vi "Gather_Deal_Data_V2_0_20160104.vi"(8 "strModelChoice":string(combo)="WD5500", 9 "写指令":bool=TRUE, 10 "1号机端口":refnum<visa-resource-name>="COM1") -> (2 "缓冲区数据":u32=284, 3 "strResultArrayOut":string[](array[string]))   [LabVIEW 2011]
uses:
  <vilib>/Instr/_visa.llb/VISA Configure Serial Port (Instr).vi
panel:
  in  "Start":bool
  out "mu08BufSize":u8
  out "mbfDealData":bool
  out "mu08SendCmd":u8=3
  in  "CmdNumCount":u8
  out "mu08ArrayBuf0":u8[](array[numeric])=[90, 165, 142, 1, 240, 0, 1, 88, 200, 2, 0, 207, 3, 0, 219, 7, 1, 40, 11, 0, 0, 12, 0, 0, 13, 0, 0, 14, 0, 0, 21, 0, 0, 22, 0, 0, 23, 0, 0, 24, 150, 154, 29, 0, 0, 0, 0, 31, 0, 0, 33, 0, 34, 1, 64, 35, 0, 41, 0, 42, 0, 43, 0, 44, 12, 158, 45, 0, 0, 46, 0, 240, 47, 240, 48, 0, 49, 0, 50, 136, 51, 0, 52, 0, 53, 0, 54, 132, 58, 0, 59, 0, 60, 241, 61, 32, 32, 32, 32, 82, 64, 73, 83, 90, 2, 4, 0, 2, 4, 0, 0, 0, 0, 2, 0, 0, 0, 104, 201, 113, 49, 49, 53, 202, 70, 52, 48, 53, 203, 57, 48, 48, 66, 204, 32, 32, 48, 53, 251, 6, 87, 112, 90, 165, 142, 1, 240, 0, 1, 88, 200, 2, 0, 207, 3, 0, 219, 7, 1, 40, 11, 0, 0, 12, 0, 0, 13, 0, 0, 14, 0, 0, 21, 0, 0, 22, 0, 0, 23, 0, 0, 24, 150, 151, 29, 0, 0, 0, 0, 31, 0, 0, 33, 0, 34, 1, 64, 35, 0, 41, 0, 42, 0, 43, 0, 44, 12, 158, 45, 0, 0, 46, 0, 240, 47, 240, 48, 0, 49, 0, 50, 136, 51, 0, 52, 0, 53, 0, 54, 132, 58, 0, 59, 0, 60, 241, 61, 32, 32, 32, 32, 82, 64, 73, 83, 90, 2, 4, 0, 2, 4, 0, 0, 0, 0, 2, 0, 0, 0, 104, 201, 113, 49, 49, 53, 202, 70, 52, 48, 53, 203, 57, 48, 48, 66, 204, 32, 32, 48, 53, 251, 6, 95, 118] format="0x%x"
  out "mu16ArrayBuf0":u16=284
  out "mu08ArrayDatas":u8[](array[numeric])=[90, 165, 142, 1, 240, 0, 1, 88, 200, 2, 0, 207, 3, 0, 219, 7, 1, 40, 11, 0, 0, 12, 0, 0, 13, 0, 0, 14, 0, 0, 21, 0, 0, 22, 0, 0, 23, 0, 0, 24, 150, 154, 29, 0, 0, 0, 0, 31, 0, 0, 33, 0, 34, 1, 64, 35, 0, 41, 0, 42, 0, 43, 0, 44, 12, 158, 45, 0, 0, 46, 0, 240, 47, 240, 48, 0, 49, 0, 50, 136, 51, 0, 52, 0, 53, 0, 54, 132, 58, 0, 59, 0, 60, 241, 61, 32, 32, 32, 32, 82, 64, 73, 83, 90, 2, 4, 0, 2, 4, 0, 0, 0, 0, 2, 0, 0, 0, 104, 201, 113, 49, 49, 53, 202, 70, 52, 48, 53, 203, 57, 48, 48, 66, 204, 32, 32, 48, 53, 251, 6, 87, 112] format="0x%x"
  out "mu08ArrayDatasSize":u16=142
  out "命令":string
  in  "mbfUartClearOne":bool=TRUE
  out "Time":u32=400
  in  "Start_2":bool
  in  "CmdNumCount 2":u8
  out "strResultArrayOut 2":string[](array[string])
  out "mbfDealData 2":bool
  out "mu08SendCmd_2":u8=3
  in  "写指令_2":bool=TRUE
  out "Time_2":u32=400
  out "缓冲区数据_2":u32=284
  out "mu08ArrayBuf0 2":u8[](array[numeric])=[90, 165, 142, 1, 240, 0, 1, 88, 200, 2, 0, 207, 3, 0, 219, 7, 1, 40, 11, 0, 0, 12, 0, 0, 13, 0, 0, 14, 0, 0, 21, 0, 0, 22, 0, 0, 23, 0, 0, 24, 150, 154, 29, 0, 0, 0, 0, 31, 0, 0, 33, 0, 34, 1, 64, 35, 0, 41, 0, 42, 0, 43, 0, 44, 12, 158, 45, 0, 0, 46, 0, 240, 47, 240, 48, 0, 49, 0, 50, 136, 51, 0, 52, 0, 53, 0, 54, 132, 58, 0, 59, 0, 60, 241, 61, 32, 32, 32, 32, 82, 64, 73, 83, 90, 2, 4, 0, 2, 4, 0, 0, 0, 0, 2, 0, 0, 0, 104, 201, 113, 49, 49, 53, 202, 70, 52, 48, 53, 203, 57, 48, 48, 66, 204, 32, 32, 48, 53, 251, 6, 87, 112, 90, 165, 142, 1, 240, 0, 1, 88, 200, 2, 0, 207, 3, 0, 219, 7, 1, 40, 11, 0, 0, 12, 0, 0, 13, 0, 0, 14, 0, 0, 21, 0, 0, 22, 0, 0, 23, 0, 0, 24, 150, 151, 29, 0, 0, 0, 0, 31, 0, 0, 33, 0, 34, 1, 64, 35, 0, 41, 0, 42, 0, 43, 0, 44, 12, 158, 45, 0, 0, 46, 0, 240, 47, 240, 48, 0, 49, 0, 50, 136, 51, 0, 52, 0, 53, 0, 54, 132, 58, 0, 59, 0, 60, 241, 61, 32, 32, 32, 32, 82, 64, 73, 83, 90, 2, 4, 0, 2, 4, 0, 0, 0, 0, 2, 0, 0, 0, 104, 201, 113, 49, 49, 53, 202, 70, 52, 48, 53, 203, 57, 48, 48, 66, 204, 32, 32, 48, 53, 251, 6, 95, 118] format="0x%x"
  out "mu16ArrayBuf0_2":u16=284
  out "mu08ArrayDatas_2":u8[](array[numeric])=[90, 165, 142, 1, 240, 0, 1, 88, 200, 2, 0, 207, 3, 0, 219, 7, 1, 40, 11, 0, 0, 12, 0, 0, 13, 0, 0, 14, 0, 0, 21, 0, 0, 22, 0, 0, 23, 0, 0, 24, 150, 154, 29, 0, 0, 0, 0, 31, 0, 0, 33, 0, 34, 1, 64, 35, 0, 41, 0, 42, 0, 43, 0, 44, 12, 158, 45, 0, 0, 46, 0, 240, 47, 240, 48, 0, 49, 0, 50, 136, 51, 0, 52, 0, 53, 0, 54, 132, 58, 0, 59, 0, 60, 241, 61, 32, 32, 32, 32, 82, 64, 73, 83, 90, 2, 4, 0, 2, 4, 0, 0, 0, 0, 2, 0, 0, 0, 104, 201, 113, 49, 49, 53, 202, 70, 52, 48, 53, 203, 57, 48, 48, 66, 204, 32, 32, 48, 53, 251, 6, 87, 112] format="0x%x"
  out "mu08ArrayDatasSize_2":u16=142
  out "mu08BufSize_2":u8
  in  "strModelChoice_2":string(combo)="WD5500"
  out "命令_2":string
  in  "mbfUartClearOne 2":bool=TRUE
  in  "2号机端口":refnum<visa-resource-name>="COM3"
  in  "Start_3":bool
  out "命令_3":string
  in  "CmdNumCount_3":u8
  out "mu16ArrayBuf0_3":u16=284
  out "mu08ArrayDatasSize_3":u16=142
  out "mu08BufSize_3":u8
  out "mu08ArrayBuf0_3":u8[](array[numeric])=[90, 165, 142, 1, 240, 0, 1, 88, 200, 2, 0, 207, 3, 0, 219, 7, 1, 40, 11, 0, 0, 12, 0, 0, 13, 0, 0, 14, 0, 0, 21, 0, 0, 22, 0, 0, 23, 0, 0, 24, 150, 154, 29, 0, 0, 0, 0, 31, 0, 0, 33, 0, 34, 1, 64, 35, 0, 41, 0, 42, 0, 43, 0, 44, 12, 158, 45, 0, 0, 46, 0, 240, 47, 240, 48, 0, 49, 0, 50, 136, 51, 0, 52, 0, 53, 0, 54, 132, 58, 0, 59, 0, 60, 241, 61, 32, 32, 32, 32, 82, 64, 73, 83, 90, 2, 4, 0, 2, 4, 0, 0, 0, 0, 2, 0, 0, 0, 104, 201, 113, 49, 49, 53, 202, 70, 52, 48, 53, 203, 57, 48, 48, 66, 204, 32, 32, 48, 53, 251, 6, 87, 112, 90, 165, 142, 1, 240, 0, 1, 88, 200, 2, 0, 207, 3, 0, 219, 7, 1, 40, 11, 0, 0, 12, 0, 0, 13, 0, 0, 14, 0, 0, 21, 0, 0, 22, 0, 0, 23, 0, 0, 24, 150, 151, 29, 0, 0, 0, 0, 31, 0, 0, 33, 0, 34, 1, 64, 35, 0, 41, 0, 42, 0, 43, 0, 44, 12, 158, 45, 0, 0, 46, 0, 240, 47, 240, 48, 0, 49, 0, 50, 136, 51, 0, 52, 0, 53, 0, 54, 132, 58, 0, 59, 0, 60, 241, 61, 32, 32, 32, 32, 82, 64, 73, 83, 90, 2, 4, 0, 2, 4, 0, 0, 0, 0, 2, 0, 0, 0, 104, 201, 113, 49, 49, 53, 202, 70, 52, 48, 53, 203, 57, 48, 48, 66, 204, 32, 32, 48, 53, 251, 6, 95, 118] format="0x%x"
  out "缓冲区数据_3":u32=284
  out "mu08ArrayDatas_3":u8[](array[numeric])=[90, 165, 142, 1, 240, 0, 1, 88, 200, 2, 0, 207, 3, 0, 219, 7, 1, 40, 11, 0, 0, 12, 0, 0, 13, 0, 0, 14, 0, 0, 21, 0, 0, 22, 0, 0, 23, 0, 0, 24, 150, 154, 29, 0, 0, 0, 0, 31, 0, 0, 33, 0, 34, 1, 64, 35, 0, 41, 0, 42, 0, 43, 0, 44, 12, 158, 45, 0, 0, 46, 0, 240, 47, 240, 48, 0, 49, 0, 50, 136, 51, 0, 52, 0, 53, 0, 54, 132, 58, 0, 59, 0, 60, 241, 61, 32, 32, 32, 32, 82, 64, 73, 83, 90, 2, 4, 0, 2, 4, 0, 0, 0, 0, 2, 0, 0, 0, 104, 201, 113, 49, 49, 53, 202, 70, 52, 48, 53, 203, 57, 48, 48, 66, 204, 32, 32, 48, 53, 251, 6, 87, 112] format="0x%x"
  in  "strModelChoice 2":string(combo)="WD5500"
  in  "写指令_3":bool=TRUE
  in  "3号机端口":refnum<visa-resource-name>="COM3"
  in  "mbfUartClearOne_3":bool=TRUE
  out "mbfDealData_3":bool
  out "Time_3":u32=400
  out "strResultArrayOut_3":string[](array[string])
  out "mu08SendCmd_2 2":u8=3
  in  "Start_4":bool
  in  "strModelChoice_4":string(combo)="WD5500"
  out "Time_4":u32=400
  out "mbfDealData_4":bool
  in  "mbfUartClearOne_4":bool=TRUE
  out "strResultArrayOut_4":string[](array[string])
  out "mu08SendCmd_4":u8=3
  out "命令_4":string
  in  "写指令_4":bool=TRUE
  out "mu08ArrayDatas_4":u8[](array[numeric])=[90, 165, 142, 1, 240, 0, 1, 88, 200, 2, 0, 207, 3, 0, 219, 7, 1, 40, 11, 0, 0, 12, 0, 0, 13, 0, 0, 14, 0, 0, 21, 0, 0, 22, 0, 0, 23, 0, 0, 24, 150, 154, 29, 0, 0, 0, 0, 31, 0, 0, 33, 0, 34, 1, 64, 35, 0, 41, 0, 42, 0, 43, 0, 44, 12, 158, 45, 0, 0, 46, 0, 240, 47, 240, 48, 0, 49, 0, 50, 136, 51, 0, 52, 0, 53, 0, 54, 132, 58, 0, 59, 0, 60, 241, 61, 32, 32, 32, 32, 82, 64, 73, 83, 90, 2, 4, 0, 2, 4, 0, 0, 0, 0, 2, 0, 0, 0, 104, 201, 113, 49, 49, 53, 202, 70, 52, 48, 53, 203, 57, 48, 48, 66, 204, 32, 32, 48, 53, 251, 6, 87, 112] format="0x%x"
  in  "CmdNumCount_4":u8
  out "缓冲区数据_4":u32=284
  out "mu08BufSize_4":u8
  out "mu08ArrayBuf0_4":u8[](array[numeric])=[90, 165, 142, 1, 240, 0, 1, 88, 200, 2, 0, 207, 3, 0, 219, 7, 1, 40, 11, 0, 0, 12, 0, 0, 13, 0, 0, 14, 0, 0, 21, 0, 0, 22, 0, 0, 23, 0, 0, 24, 150, 154, 29, 0, 0, 0, 0, 31, 0, 0, 33, 0, 34, 1, 64, 35, 0, 41, 0, 42, 0, 43, 0, 44, 12, 158, 45, 0, 0, 46, 0, 240, 47, 240, 48, 0, 49, 0, 50, 136, 51, 0, 52, 0, 53, 0, 54, 132, 58, 0, 59, 0, 60, 241, 61, 32, 32, 32, 32, 82, 64, 73, 83, 90, 2, 4, 0, 2, 4, 0, 0, 0, 0, 2, 0, 0, 0, 104, 201, 113, 49, 49, 53, 202, 70, 52, 48, 53, 203, 57, 48, 48, 66, 204, 32, 32, 48, 53, 251, 6, 87, 112, 90, 165, 142, 1, 240, 0, 1, 88, 200, 2, 0, 207, 3, 0, 219, 7, 1, 40, 11, 0, 0, 12, 0, 0, 13, 0, 0, 14, 0, 0, 21, 0, 0, 22, 0, 0, 23, 0, 0, 24, 150, 151, 29, 0, 0, 0, 0, 31, 0, 0, 33, 0, 34, 1, 64, 35, 0, 41, 0, 42, 0, 43, 0, 44, 12, 158, 45, 0, 0, 46, 0, 240, 47, 240, 48, 0, 49, 0, 50, 136, 51, 0, 52, 0, 53, 0, 54, 132, 58, 0, 59, 0, 60, 241, 61, 32, 32, 32, 32, 82, 64, 73, 83, 90, 2, 4, 0, 2, 4, 0, 0, 0, 0, 2, 0, 0, 0, 104, 201, 113, 49, 49, 53, 202, 70, 52, 48, 53, 203, 57, 48, 48, 66, 204, 32, 32, 48, 53, 251, 6, 95, 118] format="0x%x"
  in  "4号机端口":refnum<visa-resource-name>="COM3"
  out "mu08ArrayDatasSize_4":u16=142
  out "mu16ArrayBuf0_4":u16=284
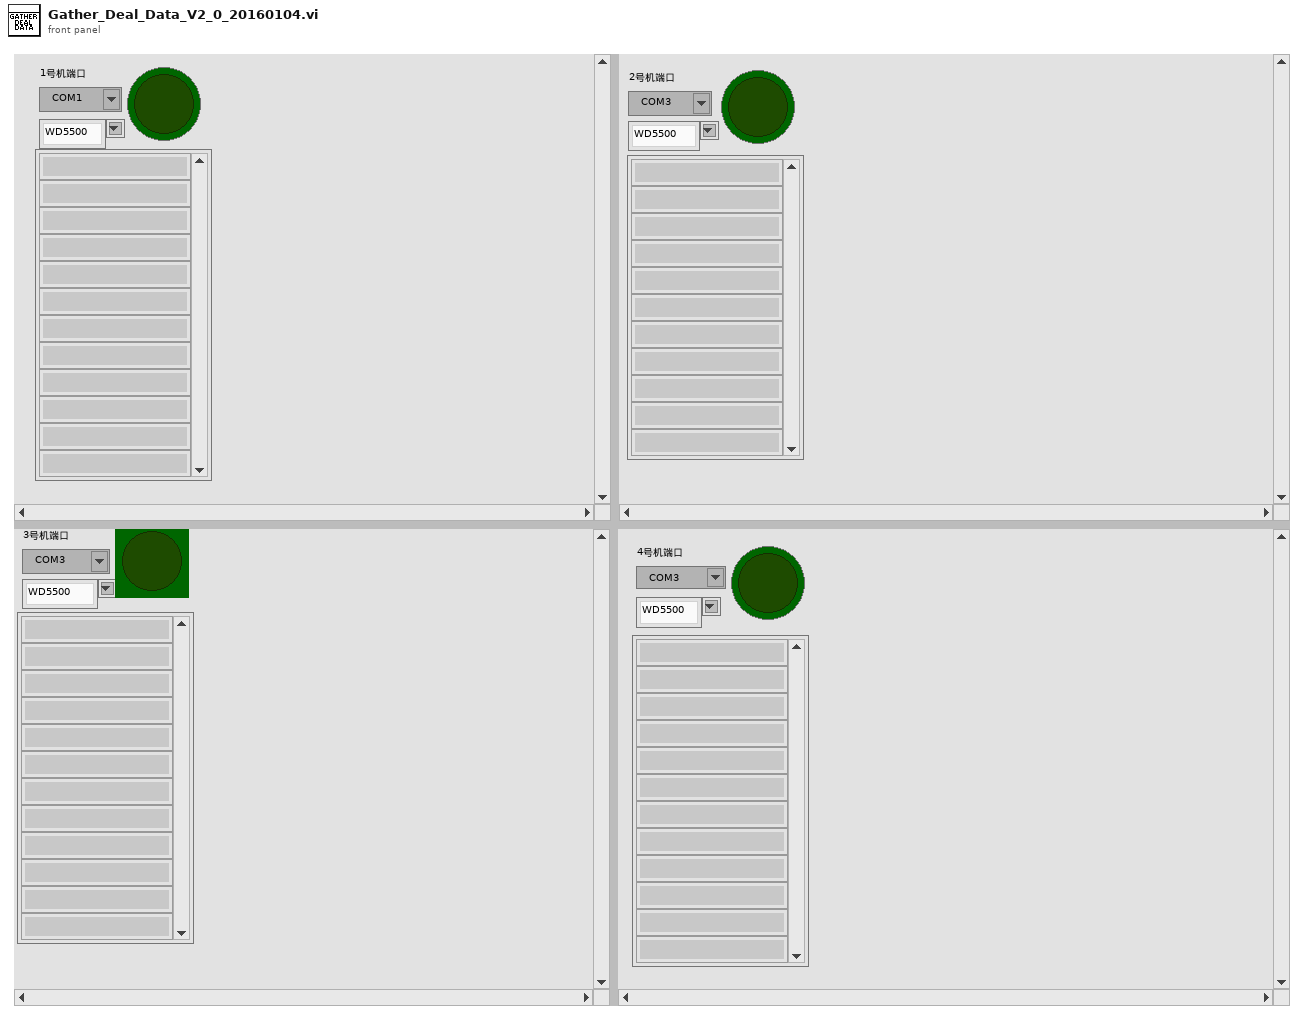
[diagram p1: front panel]
types:
  T1 = enum16{"open", "replace", "create", "open or create", "replace or create", "replace or create with confirmation"}
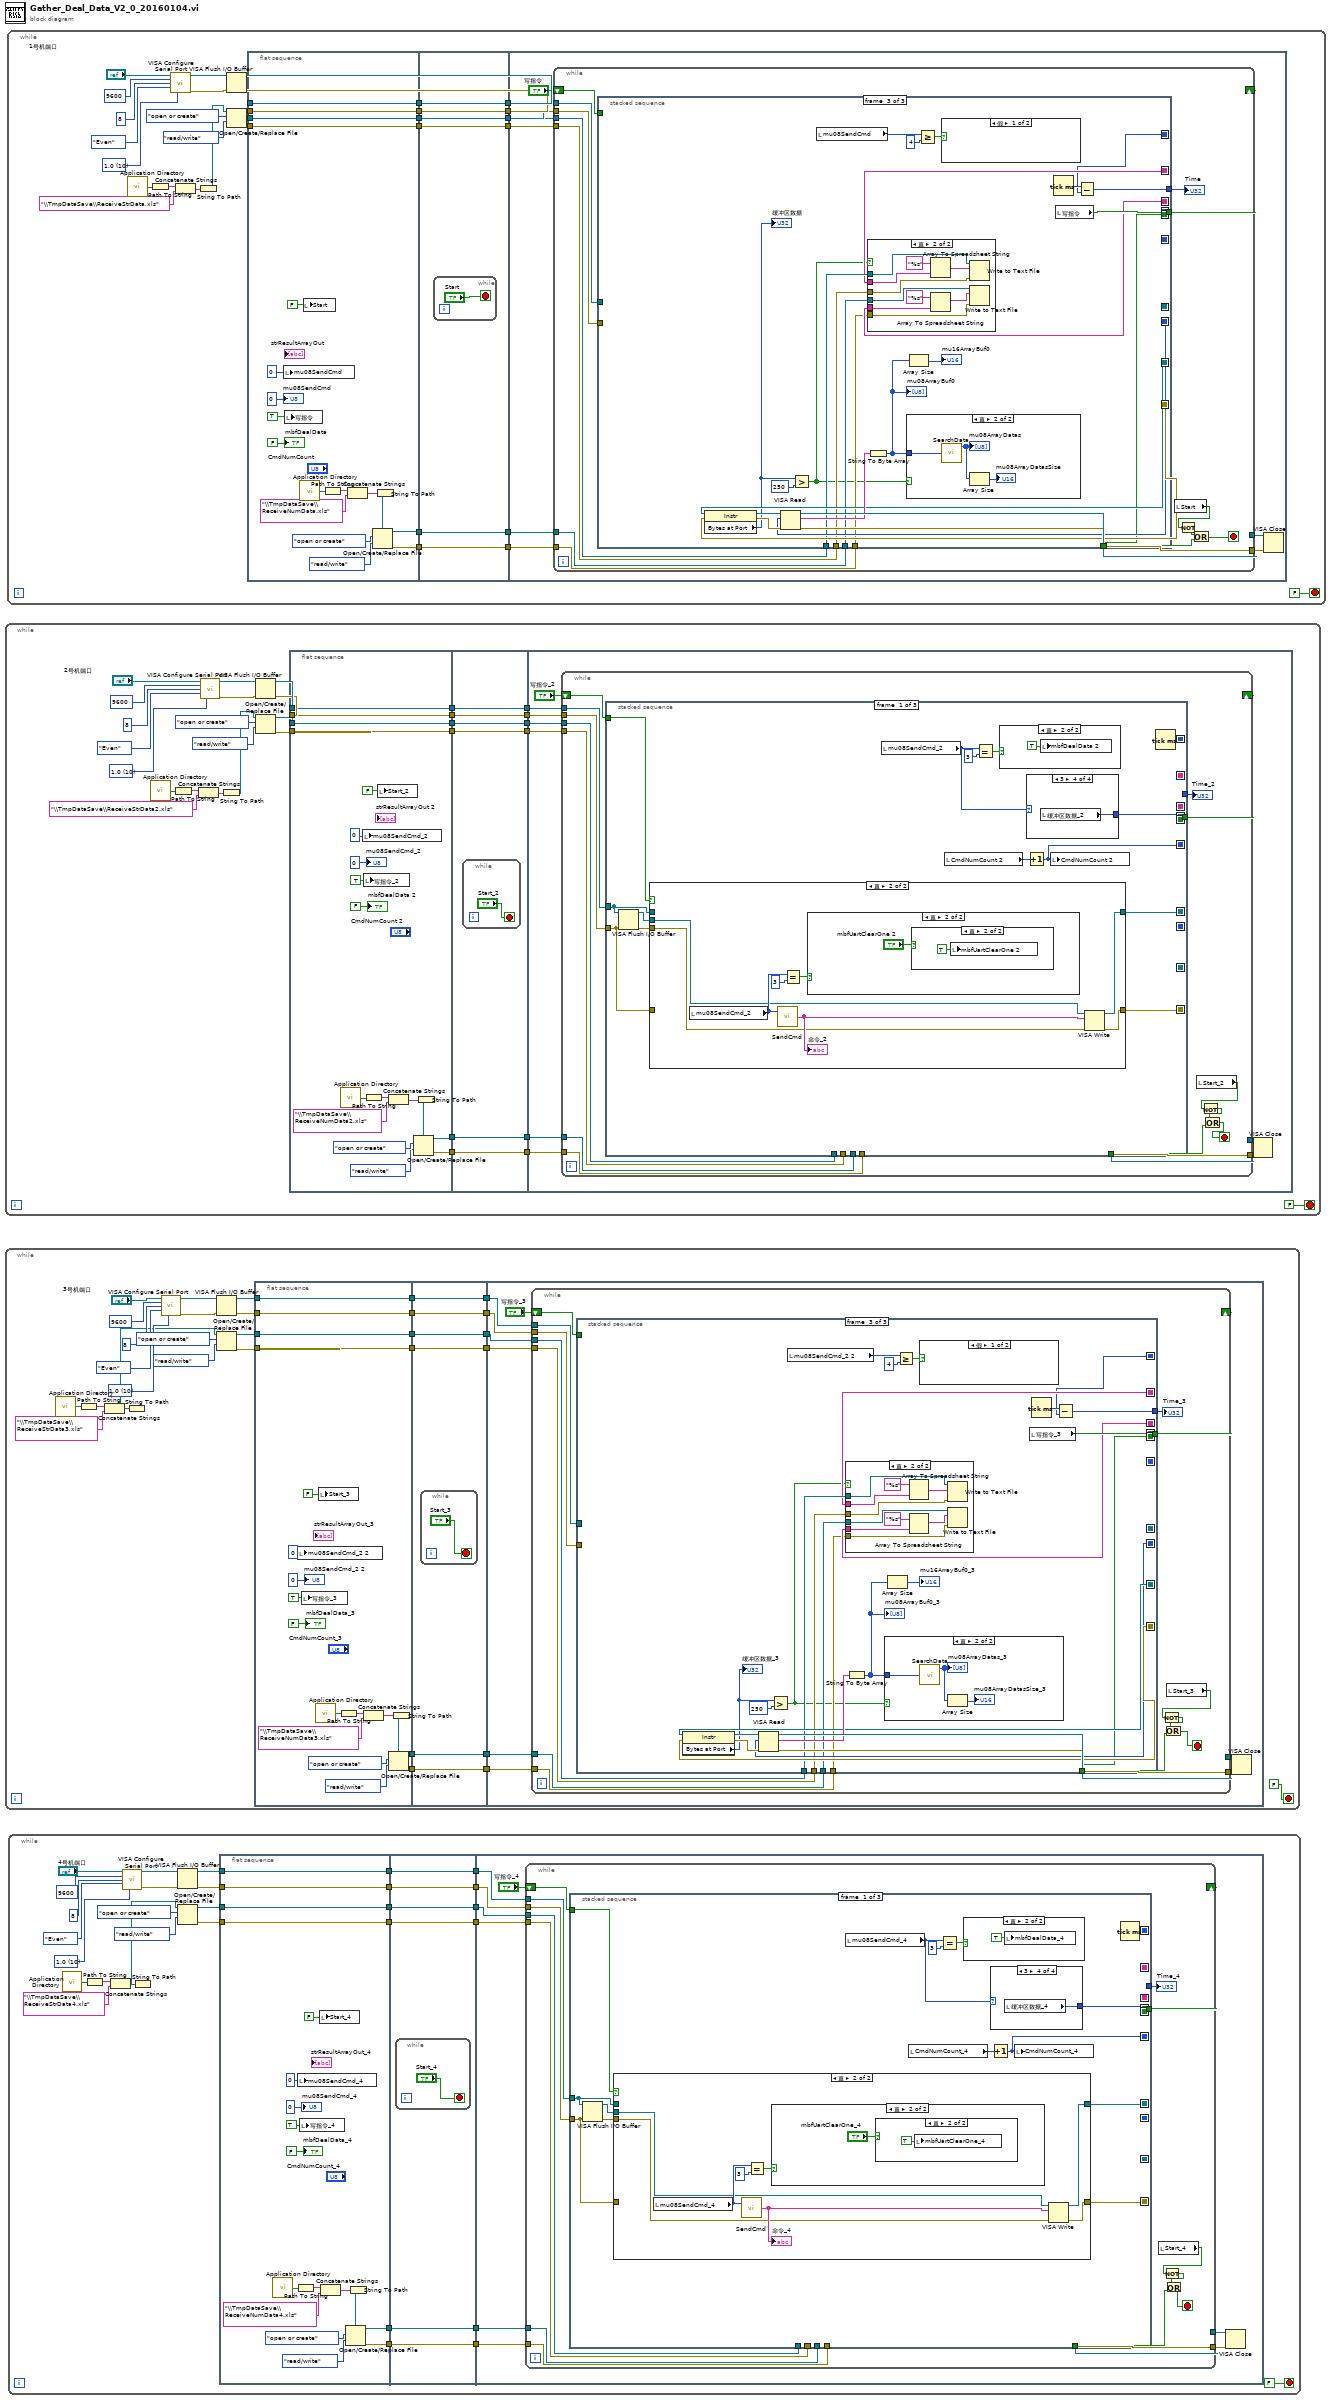
[diagram p0: block diagram]
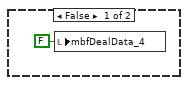
[diagram p2: hidden frame]
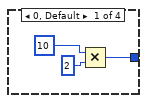
[diagram p3: hidden frame]
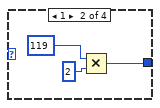
[diagram p4: hidden frame]
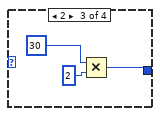
[diagram p5: hidden frame]
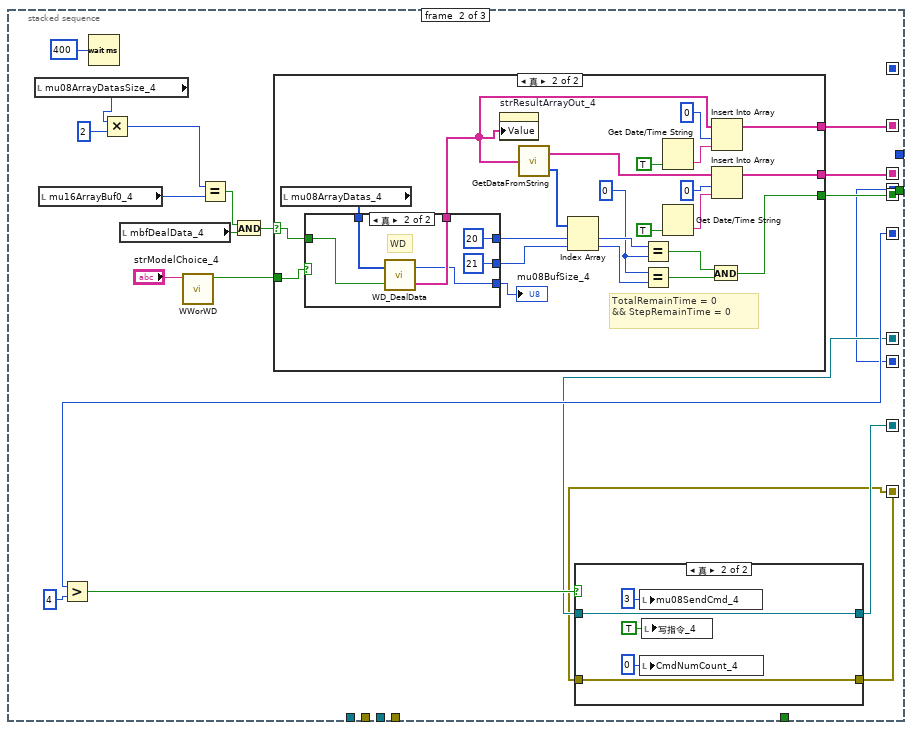
[diagram p9: hidden frame]
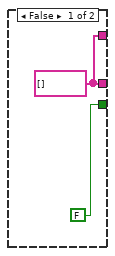
[diagram p10: hidden frame]
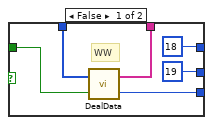
[diagram p11: hidden frame]
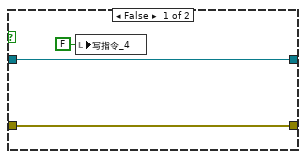
[diagram p12: hidden frame]
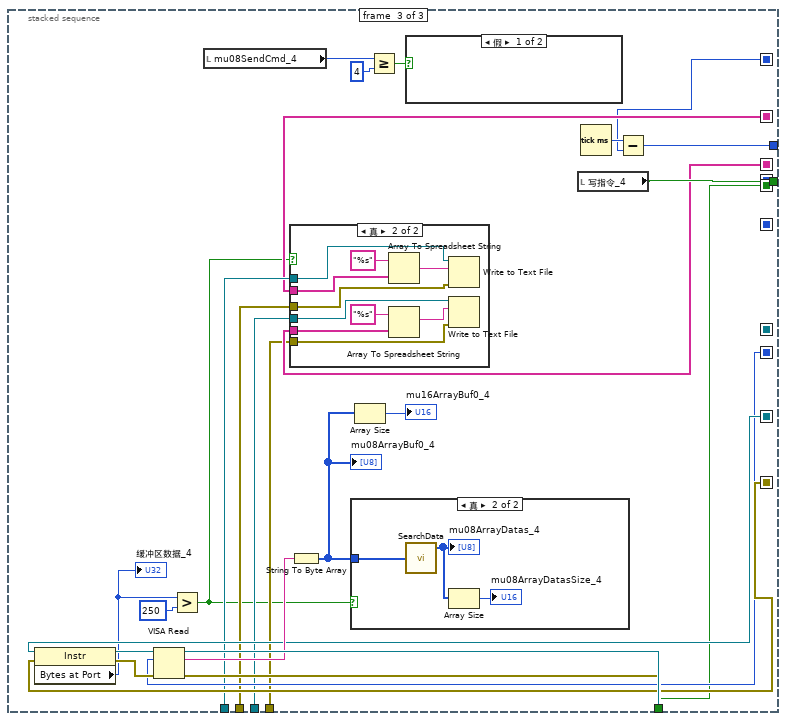
[diagram p13: hidden frame]
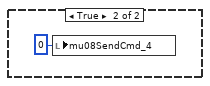
[diagram p16: hidden frame]
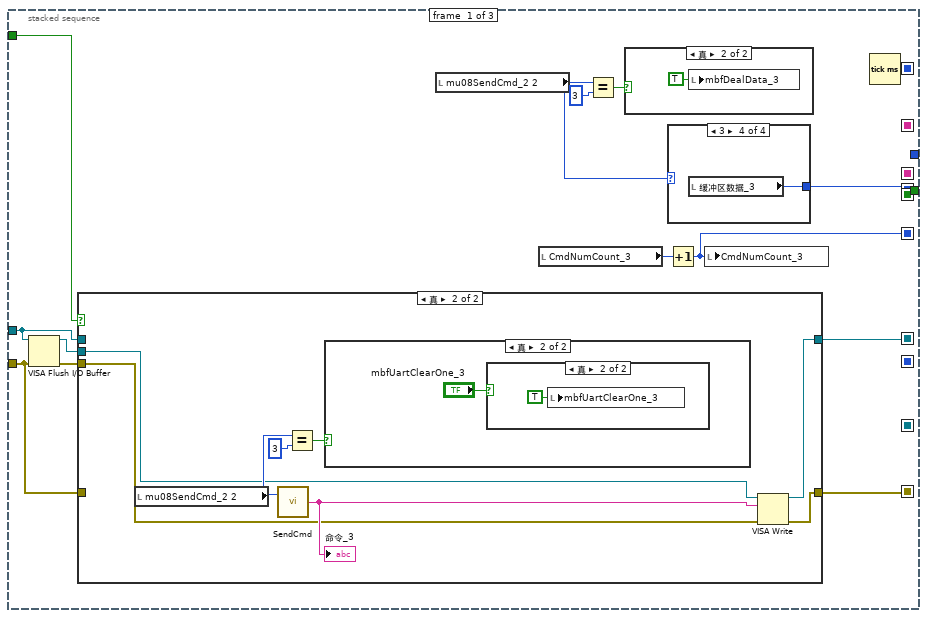
[diagram p17: hidden frame]
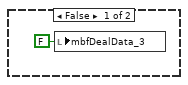
[diagram p18: hidden frame]
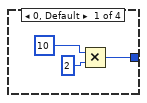
[diagram p19: hidden frame]
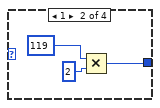
[diagram p20: hidden frame]
diagram:
  n1 = while {
    stop <- FALSE stop-if-true
    w15 = u16 10 items=["1.0"=10, "1.5"=15, "2.0"=20] ("stop bits (10: 1 bit)")
    n2 = call <vilib>:"Application Directory.vi"() -> ("Application Directory"=w5:path)
    n3 = Path To String(path=w5) -> (string=w4:string)
    n4 = Concatenate Strings(w4, "\\TmpDataSave\\ReceiveStrData2.xls" ("字符串")) -> (w2:string)
    n5 = call-poly "VISA Configure Serial Port"("VISA resource name"="2号机端口", "baud rate (9600)"=u32 9600, "data bits (8)"=u16 8, "parity (0:none)"=enum16{"None", "Odd", "Even", "Mark", "Space"}."Even", "stop bits (10: 1 bit)"=w15) -> ("VISA resource name out"=w14:refnum<visa-resource-name>, "error out"=w13:errorcluster)  [unwired: 9 in]
    n6 = String To Path(string=w2) -> (path=w8:path)
    n7 = VISA Flush I/O Buffer(VISA resource name=w14, error in (no error)=w13) -> (VISA resource name out=w12:refnum<visa-resource-name>, error out=w11:errorcluster)  [unwired: 1 in]
    n8 = Open/Create/Replace File(file path (use dialog)=w8, operation (0:open)=T1."open or create" ("操作(0:open)"), access (0:read/write)=enum16{"read/write", "read-only", "write-only"}."read/write" ("权限(0:read/write)")) -> (refnum out=w7:refnum<file>, error out=w6:errorcluster)  [unwired: 3 in, 1 out]
    n9 = flat-sequence {
      tunnel: w6 -> [w46]
      tunnel: w7 -> [w47]
      tunnel: w11 -> [w48]
      tunnel: w12 -> [w49]
      tunnel: [w49] -> w31
      tunnel: [w48] -> w30
      tunnel: [w47] -> w29
      tunnel: [w46] -> w28
      tunnel: [w33] -> w27
      tunnel: [w32] -> w26
      tunnel: [w55] -> w25
      tunnel: [w54] -> w24
      tunnel: [w53] -> w23
      tunnel: [w52] -> w22
      tunnel: [w51] -> w21
      tunnel: [w50] -> w20
      tunnel: w31 -> [w55]
      tunnel: w30 -> [w54]
      tunnel: w29 -> [w53]
      tunnel: w28 -> [w52]
      tunnel: w27 -> [w50]
      tunnel: w26 -> [w51]
      tunnel: w25 -> [w62]
      tunnel: w24 -> [w61]
      tunnel: w23 -> [w60]
      tunnel: w22 -> [w59]
      tunnel: w21 -> [w58]
      tunnel: w20 -> [w57]
      frame #0 {
        n10 = call <vilib>:"Application Directory.vi"() -> ("Application Directory"=w37:path)
        n11 = local write "mu08SendCmd_2"(u8 0 ("Cmd值")) -> ()
        n12 = local write "写指令_2"(TRUE ("写指令")) -> ()
        n13 = Path To String(path=w37) -> (string=w38:string)
        n14 = local write "Start_2"(FALSE ("Start_2")) -> ()
        n15 = Concatenate Strings(w38, "\\TmpDataSave\\ReceiveNumData2.xls" ("字符串")) -> (w40:string)
        n16 = String To Path(string=w40) -> (path=w36:path)
        n17 = Open/Create/Replace File(file path (use dialog)=w36, operation (0:open)=T1."open or create" ("操作(0:open)"), access (0:read/write)=enum16{"read/write", "read-only", "write-only"}."read/write" ("权限(0:read/write)")) -> (refnum out=w33:refnum<file>, error out=w32:errorcluster)  [unwired: 3 in, 1 out]
        "mu08SendCmd_2" <- u8 0 ("mu08SendCmd")
        "mbfDealData 2" <- FALSE ("mbfDealData")
      }
      frame #1 {
        n18 = while {
          stop <- "Start_2" stop-if-true
        }
      }
      frame #2 {
        n19 = while {
          tunnel: w62 -> [w80]
          tunnel: w61 -> [w79]
          tunnel: [w78] -> w65
          tunnel: [w77] -> w64
          shift-right: [w75] -> _
          shift-left: "写指令_2" -> [w76]
          tunnel: w60 -> [w74]
          tunnel: w59 -> [w73]
          tunnel: w58 -> [w71]
          tunnel: w57 -> [w70]
          stop <- w66 stop-if-true
          n20 = stacked-sequence {
            seq-local: [w94 _ _] -> [_ w134 _]
            seq-local: [w93 _ _] -> [_ w133 _]
            seq-local: [w90 _ _] -> [_ w137 _]
            seq-local: [w81 _ _] -> [_ w121 _]
            seq-local: [w82 _ _] -> [_ w131 _]
            seq-local: [_ w136 _] -> [_ _ w207]
            seq-local: [_ w135 _] -> [_ _ w206]
            seq-local: [_ w132 _] -> [_ _ w197]
            seq-local: [_ w131 _] -> [_ _ w195]
            seq-local: [_ w130 _] -> [_ _ w193]
            seq-local: [_ w125 _] -> [_ _ w186]
            seq-local: [_ w121 _] -> [_ _ w202]
            tunnel: w80 -> [w86 _ _]
            tunnel: w79 -> [w85 _ _]
            tunnel: w76 -> [w92 _ _]
            tunnel: [_ _ w210] -> w78
            tunnel: [_ _ w209] -> w77
            tunnel: [_ _ w201] -> w75
            tunnel: w74 -> [_ _ w199]
            tunnel: w73 -> [_ _ w198]
            tunnel: [_ _ w194] -> w72
            tunnel: w71 -> [_ _ w192]
            tunnel: w70 -> [_ _ w191]
            tunnel: [_ _ w186] -> w67
            frame #0 {
              n21 = VISA Flush I/O Buffer(VISA resource name=w86, error in (no error)=w85) -> (VISA resource name out=w83:refnum<visa-resource-name>, error out=w84:errorcluster)  [unwired: 1 in]
              n22 = case shown="真" w92 {
                tunnel: w86 -> [w108 _]
                tunnel: w85 -> [w107 _]
                tunnel: [w108 w116] -> w94
                tunnel: [w107 w115] -> w93
                tunnel: w84 -> [_ w110]
                tunnel: w83 -> [_ w109]
                frame False {
                }
                frame True {
                  n23 = local read "mu08SendCmd_2"() -> (w112:u8)
                  n24 = call "SendCmd.vi"("索引 (行)"=w112) -> ("字符串"=w114:string)  [unwired: 1 in]
                  "命令_2" <- w114
                  n25 = Equal?(x=w112, y=u8 3) -> (x = y?=w111:bool)
                  n26 = case shown="真" w111 {
                    frame False {
                    }
                    frame True {
                      n27 = case shown="真" "mbfUartClearOne 2" {
                        frame False {
                        }
                        frame True {
                          n28 = local write "mbfUartClearOne 2"(TRUE ("mbfUartClearOne")) -> ()
                        }
                      }
                    }
                  }
                  n29 = VISA Write(VISA resource name=w109, write buffer=w114, error in (no error)=w110) -> (VISA resource name out=w116:refnum<visa-resource-name>, error out=w115:errorcluster)  [unwired: 1 out]
                }
              }
              n30 = local read "mu08SendCmd_2"() -> (w89:u8)
              n31 = local read "CmdNumCount 2"() -> (w91:u8)
              n32 = Equal?(x=w89, y=u8 3) -> (x = y?=w87:bool)
              n33 = case shown="真" w87 {
                frame False {
                  n34 = local write "mbfDealData 2"(FALSE ("mbfDealData")) -> ()
                }
                frame True {
                  n35 = local write "mbfDealData 2"(TRUE ("mbfDealData")) -> ()
                }
              }
              n36 = case shown="3" w89 {
                tunnel: [w97 w100 w103 w106] -> w81
                frame 0, Default {
                  n37 = Multiply(x=10, y=2) -> (x*y=w97:i32)
                }
                frame 1 {
                  n38 = Multiply(x=119, y=2) -> (x*y=w100:i32)
                }
                frame 2 {
                  n39 = Multiply(x=30, y=2) -> (x*y=w103:i32)
                }
                frame 3 {
                  n40 = local read "缓冲区数据_2"() -> (w106:u32)
                }
              }
              n41 = Increment(x=w91) -> (x+1=w90:u8)
              n42 = local write "CmdNumCount 2"(w90) -> ()
              n43 = Tick Count (ms)() -> (millisecond timer value=w82:u32)
            }
            frame #1 {
              n44 = local read "mu08ArrayDatasSize_2"() -> (w124:u16)
              n45 = local read "mu16ArrayBuf0_2"() -> (w129:u16)
              n46 = Greater?(x=w137, y=u8 4) -> (0:w138:bool)
              n47 = Wait (ms)(milliseconds to wait=u32 400 ("等待时间（毫秒）")) -> ()  [unwired: 1 out]
              n48 = Multiply(x=w124, y=u8 2) -> (x*y=w122:u16)
              n49 = local read "mbfDealData 2"() -> (w128:bool)
              n50 = call "WWorWD.vi"("strModelChoice"="strModelChoice_2") -> ("WWorWD"=w119:bool)  [unwired: 9 in, 1 out]
              n51 = Equal?(x=w122, y=w129) -> (x = y?=w127:bool)
              n52 = And(x=w127, y=w128) -> (x .and. y?=w126:bool)
              n53 = case shown="真" w126 {
                selector: w126 -> [_ w145]
                tunnel: [w142 w163] -> w132
                tunnel: [w142 w158] -> w130
                tunnel: [FALSE w150] -> w125
                tunnel: w119 -> [_ w146]
                frame False {
                  w142 = string[] []
                }
                frame True {
                  w154 = u32 0 ("y")
                  # "TotalRemainTime = 0\n&& StepRemainTime = 0"
                  n54 = local read "mu08ArrayDatas_2"() -> (w149:u8[])
                  n55 = case shown="真" w146 {
                    tunnel: [w171 w177] -> w143
                    tunnel: [w170 w176] -> w144
                    tunnel: w149 -> [w169 w175]
                    tunnel: [18 ("索引") 20 ("索引")] -> w148
                    tunnel: [19 ("索引") 21 ("索引")] -> w147
                    tunnel: w145 -> [w166 w172]
                    frame False {
                      # "WW"
                      n56 = call "DealData.vi"("mbfDealData"=w166, "ArrayIn"=w169) -> ("mu08BufSize"=w170:u8, "Result"=w171:string[])
                    }
                    frame True {
                      # "WD"
                      n57 = call "WD_DealData.vi"("mbfDealData"=w172, "ArrayIn"=w175) -> ("ResultArrayOut"=w177:string[], "mu08BufSize"=w176:u8)
                    }
                  }
                  "mu08BufSize_2" <- w144
                  n58 = property on="strResultArrayOut 2" class="Arr (严格)"("Value"=w143) -> ()  [unwired: 2 in, 2 out]
                  n59 = call "GetDataFromString.vi"("strArrayIn"=w143) -> ("strArrayBuf"=w157:string[], "mu32ArrayOut"=w156:u32[])
                  n60 = Index Array(array=w156, index #1=w148, index #2=w147) -> (element #1=w155:u32, element #2=w153:u32)
                  n61 = Equal?(x=w155, y=w154) -> (x = y?=w152:bool)
                  n62 = Equal?(x=w154, y=w153) -> (x = y?=w151:bool)
                  n63 = Get Date/Time String(want seconds? (F)=TRUE ("需要秒？(F)")) -> (time string=w164:string)  [unwired: 2 in, 1 out]
                  n64 = Get Date/Time String(want seconds? (F)=TRUE ("需要秒？(F)")) -> (time string=w160:string)  [unwired: 2 in, 1 out]
                  n65 = And(x=w152, y=w151) -> (x .and. y?=w150:bool)
                  n66 = Insert Into Array(array=w143, index=0 ("索引"), new element=w164) -> (w163:string[])
                  n67 = Insert Into Array(array=w157, index=0 ("索引"), new element=w160) -> (w158:string[])
                }
              }
              n68 = case shown="真" w138 {
                tunnel: [w179 w183] -> w136
                tunnel: [w178 w182] -> w135
                tunnel: w134 -> [w179 w183]
                tunnel: w133 -> [w178 w182]
                frame False {
                  n69 = local write "写指令_2"(FALSE ("写指令")) -> ()
                }
                frame True {
                  n70 = local write "mu08SendCmd_2"(u8 3 ("mu08SendCmd")) -> ()
                  n71 = local write "CmdNumCount 2"(u8 0 ("CmdNumCount")) -> ()
                  n72 = local write "写指令_2"(TRUE ("写指令")) -> ()
                }
              }
            }
            frame #2 {
              n73 = property class="Instr"(reference=w207, error in=w206) -> (reference out=w212:refnum<visa-resource-name>, error out=w211:errorcluster, "Bytes at Port"=w189:u32)
              "缓冲区数据_2" <- w189
              n74 = VISA Read(VISA resource name=w212, byte count=w202, error in (no error)=w211) -> (VISA resource name out=w210:refnum<visa-resource-name>, read buffer=w208:string, error out=w209:errorcluster)  [unwired: 1 out]
              n75 = Greater?(x=w189, y=250) -> (0:w188:bool)
              n76 = local read "mu08SendCmd_2"() -> (w205:u8)
              n77 = case shown="真" w188 {
                tunnel: w199 -> [_ w223]
                tunnel: w198 -> [_ w222]
                tunnel: w197 -> [_ w221]
                tunnel: w193 -> [_ w220]
                tunnel: w192 -> [_ w217]
                tunnel: w191 -> [_ w216]
                frame False {
                }
                frame True {
                  n78 = Array To Spreadsheet String(array=w221, 3:"%s" ("格式字符串")) -> (spreadsheet string=w225:string)  [unwired: 1 in]
                  n79 = Array To Spreadsheet String(array=w220, 3:"%s" ("格式字符串")) -> (spreadsheet string=w218:string)  [unwired: 1 in]
                  n80 = Write to Text File(file (use dialog)=w223, text=w225, error in=w222) -> ()  [unwired: 1 in, 3 out]
                  n81 = Write to Text File(file (use dialog)=w216, text=w218, error in=w217) -> ()  [unwired: 1 in, 3 out]
                }
              }
              n82 = String To Byte Array(string=w208) -> (unsigned byte array=w187:u8[])
              "mu08ArrayBuf0 2" <- w187
              n83 = case shown="真" w188 {
                tunnel: w187 -> [_ w214]
                frame False {
                }
                frame True {
                  n84 = call "SearchData.vi"("ArrayIn"=w214) -> ("ArrayOut"=w213:u8[])  [unwired: 2 out]
                  "mu08ArrayDatas_2" <- w213
                  n85 = Array Size(array=w213) -> (size(s)=→"mu08ArrayDatasSize_2":i32)
                }
              }
              n86 = Array Size(array=w187) -> (size(s)=→"mu16ArrayBuf0_2":i32)
              n87 = Greater Or Equal?(x=w205, y=u8 4) -> (x >= y?=w203:bool)
              n88 = case shown="假" w203 {
                frame False {
                }
                frame True {
                  n89 = local write "mu08SendCmd_2"(u8 0 ("Cmd值")) -> ()
                }
              }
              n90 = local read "写指令_2"() -> (w201:bool)
              n91 = Tick Count (ms)() -> (millisecond timer value=w196:u32)
              n92 = Subtract(x=w196, y=w195) -> (x-y=w194:u32)
            }
          }
          "Time_2" <- w72
          n93 = local read "Start_2"() -> (w69:bool)
          n94 = Not(x=w69) -> (.not. x?=w68:bool)
          n95 = Or(x=w68, y=w67) -> (x .or. y?=w66:bool)
        }
        n96 = VISA Close(VISA resource name=w65, error in (no error)=w64) -> ()  [unwired: 1 out]
      }
    }
  }
  n97 = while {
    stop <- FALSE stop-if-true
    w241 = u16 10 items=["1.0"=10, "1.5"=15, "2.0"=20] ("stop bits (10: 1 bit)")
    n98 = call <vilib>:"Application Directory.vi"() -> ("Application Directory"=w231:path)
    n99 = Path To String(path=w231) -> (string=w230:string)
    n100 = Concatenate Strings(w230, "\\TmpDataSave\\ReceiveStrData3.xls" ("字符串")) -> (w228:string)
    n101 = String To Path(string=w228) -> (path=w234:path)
    n102 = call-poly "VISA Configure Serial Port"("VISA resource name"="3号机端口", "baud rate (9600)"=u32 9600, "data bits (8)"=u16 8, "parity (0:none)"=enum16{"None", "Odd", "Even", "Mark", "Space"}."Even", "stop bits (10: 1 bit)"=w241) -> ("VISA resource name out"=w240:refnum<visa-resource-name>, "error out"=w239:errorcluster)  [unwired: 9 in]
    n103 = VISA Flush I/O Buffer(VISA resource name=w240, error in (no error)=w239) -> (VISA resource name out=w238:refnum<visa-resource-name>, error out=w237:errorcluster)  [unwired: 1 in]
    n104 = Open/Create/Replace File(file path (use dialog)=w234, operation (0:open)=T1."open or create" ("操作(0:open)"), access (0:read/write)=enum16{"read/write", "read-only", "write-only"}."read/write" ("权限(0:read/write)")) -> (refnum out=w233:refnum<file>, error out=w232:errorcluster)  [unwired: 3 in, 1 out]
    n105 = flat-sequence {
      tunnel: w232 -> [w272]
      tunnel: w233 -> [w273]
      tunnel: w237 -> [w274]
      tunnel: w238 -> [w275]
      tunnel: [w275] -> w257
      tunnel: [w274] -> w256
      tunnel: [w273] -> w255
      tunnel: [w272] -> w254
      tunnel: [w259] -> w253
      tunnel: [w260] -> w252
      tunnel: [w281] -> w251
      tunnel: [w280] -> w250
      tunnel: [w279] -> w249
      tunnel: [w278] -> w248
      tunnel: [w277] -> w247
      tunnel: [w276] -> w246
      tunnel: w257 -> [w281]
      tunnel: w256 -> [w280]
      tunnel: w255 -> [w279]
      tunnel: w254 -> [w278]
      tunnel: w253 -> [w277]
      tunnel: w252 -> [w276]
      tunnel: w251 -> [w288]
      tunnel: w250 -> [w287]
      tunnel: w249 -> [w286]
      tunnel: w248 -> [w285]
      tunnel: w247 -> [w284]
      tunnel: w246 -> [w283]
      frame #0 {
        n106 = local write "mu08SendCmd_2 2"(u8 0 ("Cmd值")) -> ()
        n107 = local write "写指令_3"(TRUE ("写指令")) -> ()
        n108 = call <vilib>:"Application Directory.vi"() -> ("Application Directory"=w264:path)
        n109 = local write "Start_3"(FALSE ("Start_3")) -> ()
        n110 = Path To String(path=w264) -> (string=w265:string)
        n111 = Concatenate Strings(w265, "\\TmpDataSave\\ReceiveNumData3.xls" ("字符串")) -> (w267:string)
        n112 = String To Path(string=w267) -> (path=w263:path)
        n113 = Open/Create/Replace File(file path (use dialog)=w263, operation (0:open)=T1."open or create" ("操作(0:open)"), access (0:read/write)=enum16{"read/write", "read-only", "write-only"}."read/write" ("权限(0:read/write)")) -> (refnum out=w260:refnum<file>, error out=w259:errorcluster)  [unwired: 3 in, 1 out]
        "mu08SendCmd_2 2" <- u8 0 ("mu08SendCmd")
        "mbfDealData_3" <- FALSE ("mbfDealData")
      }
      frame #1 {
        n114 = while {
          stop <- "Start_3" stop-if-true
        }
      }
      frame #2 {
        n115 = while {
          tunnel: w288 -> [w306]
          tunnel: w287 -> [w305]
          tunnel: [w304] -> w291
          tunnel: [w303] -> w290
          shift-right: [w301] -> _
          shift-left: "写指令_3" -> [w302]
          tunnel: w286 -> [w300]
          tunnel: w285 -> [w299]
          tunnel: w284 -> [w297]
          tunnel: w283 -> [w296]
          stop <- w293 stop-if-true
          n116 = stacked-sequence {
            seq-local: [w320 _ _] -> [_ w360 _]
            seq-local: [w319 _ _] -> [_ w359 _]
            seq-local: [w316 _ _] -> [_ w363 _]
            seq-local: [w307 _ _] -> [_ w347 _]
            seq-local: [w308 _ _] -> [_ w357 _]
            seq-local: [_ w362 _] -> [_ _ w433]
            seq-local: [_ w361 _] -> [_ _ w432]
            seq-local: [_ w358 _] -> [_ _ w423]
            seq-local: [_ w357 _] -> [_ _ w421]
            seq-local: [_ w356 _] -> [_ _ w419]
            seq-local: [_ w351 _] -> [_ _ w412]
            seq-local: [_ w347 _] -> [_ _ w428]
            tunnel: w306 -> [w312 _ _]
            tunnel: w305 -> [w311 _ _]
            tunnel: w302 -> [w318 _ _]
            tunnel: [_ _ w436] -> w304
            tunnel: [_ _ w435] -> w303
            tunnel: [_ _ w427] -> w301
            tunnel: w300 -> [_ _ w425]
            tunnel: w299 -> [_ _ w424]
            tunnel: [_ _ w420] -> w298
            tunnel: w297 -> [_ _ w418]
            tunnel: w296 -> [_ _ w417]
            tunnel: [_ _ w412] -> w292
            frame #0 {
              n117 = VISA Flush I/O Buffer(VISA resource name=w312, error in (no error)=w311) -> (VISA resource name out=w309:refnum<visa-resource-name>, error out=w310:errorcluster)  [unwired: 1 in]
              n118 = case shown="真" w318 {
                tunnel: w312 -> [w334 _]
                tunnel: w311 -> [w333 _]
                tunnel: [w334 w342] -> w320
                tunnel: [w333 w341] -> w319
                tunnel: w310 -> [_ w336]
                tunnel: w309 -> [_ w335]
                frame False {
                }
                frame True {
                  n119 = local read "mu08SendCmd_2 2"() -> (w338:u8)
                  n120 = call "SendCmd.vi"("索引 (行)"=w338) -> ("字符串"=w340:string)  [unwired: 1 in]
                  "命令_3" <- w340
                  n121 = Equal?(x=w338, y=u8 3) -> (x = y?=w337:bool)
                  n122 = case shown="真" w337 {
                    frame False {
                    }
                    frame True {
                      n123 = case shown="真" "mbfUartClearOne_3" {
                        frame False {
                        }
                        frame True {
                          n124 = local write "mbfUartClearOne_3"(TRUE ("mbfUartClearOne")) -> ()
                        }
                      }
                    }
                  }
                  n125 = VISA Write(VISA resource name=w335, write buffer=w340, error in (no error)=w336) -> (VISA resource name out=w342:refnum<visa-resource-name>, error out=w341:errorcluster)  [unwired: 1 out]
                }
              }
              n126 = local read "mu08SendCmd_2 2"() -> (w315:u8)
              n127 = local read "CmdNumCount_3"() -> (w317:u8)
              n128 = Equal?(x=w315, y=u8 3) -> (x = y?=w313:bool)
              n129 = case shown="真" w313 {
                frame False {
                  n130 = local write "mbfDealData_3"(FALSE ("mbfDealData")) -> ()
                }
                frame True {
                  n131 = local write "mbfDealData_3"(TRUE ("mbfDealData")) -> ()
                }
              }
              n132 = case shown="3" w315 {
                tunnel: [w323 w326 w329 w332] -> w307
                frame 0, Default {
                  n133 = Multiply(x=10, y=2) -> (x*y=w323:i32)
                }
                frame 1 {
                  n134 = Multiply(x=119, y=2) -> (x*y=w326:i32)
                }
                frame 2 {
                  n135 = Multiply(x=30, y=2) -> (x*y=w329:i32)
                }
                frame 3 {
                  n136 = local read "缓冲区数据_3"() -> (w332:u32)
                }
              }
              n137 = Increment(x=w317) -> (x+1=w316:u8)
              n138 = local write "CmdNumCount_3"(w316) -> ()
              n139 = Tick Count (ms)() -> (millisecond timer value=w308:u32)
            }
            frame #1 {
              n140 = local read "mu08ArrayDatasSize_3"() -> (w350:u16)
              n141 = local read "mu16ArrayBuf0_3"() -> (w355:u16)
              n142 = Greater?(x=w363, y=u8 4) -> (0:w364:bool)
              n143 = Wait (ms)(milliseconds to wait=u32 400 ("等待时间（毫秒）")) -> ()  [unwired: 1 out]
              n144 = Multiply(x=w350, y=u8 2) -> (x*y=w348:u16)
              n145 = local read "mbfDealData_3"() -> (w354:bool)
              n146 = call "WWorWD.vi"("strModelChoice"="strModelChoice 2") -> ("WWorWD"=w345:bool)  [unwired: 9 in, 1 out]
              n147 = Equal?(x=w348, y=w355) -> (x = y?=w353:bool)
              n148 = And(x=w353, y=w354) -> (x .and. y?=w352:bool)
              n149 = case shown="真" w352 {
                selector: w352 -> [_ w371]
                tunnel: [w368 w389] -> w358
                tunnel: [w368 w384] -> w356
                tunnel: [FALSE w376] -> w351
                tunnel: w345 -> [_ w372]
                frame False {
                  w368 = string[] []
                }
                frame True {
                  w380 = u32 0 ("y")
                  # "TotalRemainTime = 0\n&& StepRemainTime = 0"
                  n150 = local read "mu08ArrayDatas_3"() -> (w375:u8[])
                  n151 = case shown="真" w372 {
                    tunnel: [w397 w403] -> w369
                    tunnel: [w396 w402] -> w370
                    tunnel: w375 -> [w395 w401]
                    tunnel: [18 ("索引") 20 ("索引")] -> w374
                    tunnel: [19 ("索引") 21 ("索引")] -> w373
                    tunnel: w371 -> [w392 w398]
                    frame False {
                      # "WW"
                      n152 = call "DealData.vi"("mbfDealData"=w392, "ArrayIn"=w395) -> ("mu08BufSize"=w396:u8, "Result"=w397:string[])
                    }
                    frame True {
                      # "WD"
                      n153 = call "WD_DealData.vi"("mbfDealData"=w398, "ArrayIn"=w401) -> ("ResultArrayOut"=w403:string[], "mu08BufSize"=w402:u8)
                    }
                  }
                  "mu08BufSize_3" <- w370
                  n154 = property on="strResultArrayOut_3" class="Arr (严格)"("Value"=w369) -> ()  [unwired: 2 in, 2 out]
                  n155 = call "GetDataFromString.vi"("strArrayIn"=w369) -> ("strArrayBuf"=w383:string[], "mu32ArrayOut"=w382:u32[])
                  n156 = Index Array(array=w382, index #1=w374, index #2=w373) -> (element #1=w381:u32, element #2=w379:u32)
                  n157 = Equal?(x=w381, y=w380) -> (x = y?=w378:bool)
                  n158 = Equal?(x=w380, y=w379) -> (x = y?=w377:bool)
                  n159 = Get Date/Time String(want seconds? (F)=TRUE ("需要秒？(F)")) -> (time string=w390:string)  [unwired: 2 in, 1 out]
                  n160 = Get Date/Time String(want seconds? (F)=TRUE ("需要秒？(F)")) -> (time string=w386:string)  [unwired: 2 in, 1 out]
                  n161 = And(x=w378, y=w377) -> (x .and. y?=w376:bool)
                  n162 = Insert Into Array(array=w369, index=0 ("索引"), new element=w390) -> (w389:string[])
                  n163 = Insert Into Array(array=w383, index=0 ("索引"), new element=w386) -> (w384:string[])
                }
              }
              n164 = case shown="真" w364 {
                tunnel: [w405 w409] -> w362
                tunnel: [w404 w408] -> w361
                tunnel: w360 -> [w405 w409]
                tunnel: w359 -> [w404 w408]
                frame False {
                  n165 = local write "写指令_3"(FALSE ("写指令")) -> ()
                }
                frame True {
                  n166 = local write "mu08SendCmd_2 2"(u8 3 ("mu08SendCmd")) -> ()
                  n167 = local write "CmdNumCount_3"(u8 0 ("CmdNumCount")) -> ()
                  n168 = local write "写指令_3"(TRUE ("写指令")) -> ()
                }
              }
            }
            frame #2 {
              n169 = property class="Instr"(reference=w433, error in=w432) -> (reference out=w438:refnum<visa-resource-name>, error out=w437:errorcluster, "Bytes at Port"=w415:u32)
              "缓冲区数据_3" <- w415
              n170 = VISA Read(VISA resource name=w438, byte count=w428, error in (no error)=w437) -> (VISA resource name out=w436:refnum<visa-resource-name>, read buffer=w434:string, error out=w435:errorcluster)  [unwired: 1 out]
              n171 = Greater?(x=w415, y=250) -> (0:w414:bool)
              n172 = local read "mu08SendCmd_2 2"() -> (w431:u8)
              n173 = case shown="真" w414 {
                tunnel: w425 -> [_ w449]
                tunnel: w424 -> [_ w448]
                tunnel: w423 -> [_ w447]
                tunnel: w419 -> [_ w446]
                tunnel: w418 -> [_ w443]
                tunnel: w417 -> [_ w442]
                frame False {
                }
                frame True {
                  n174 = Array To Spreadsheet String(array=w447, 3:"%s" ("格式字符串")) -> (spreadsheet string=w451:string)  [unwired: 1 in]
                  n175 = Array To Spreadsheet String(array=w446, 3:"%s" ("格式字符串")) -> (spreadsheet string=w444:string)  [unwired: 1 in]
                  n176 = Write to Text File(file (use dialog)=w449, text=w451, error in=w448) -> ()  [unwired: 1 in, 3 out]
                  n177 = Write to Text File(file (use dialog)=w442, text=w444, error in=w443) -> ()  [unwired: 1 in, 3 out]
                }
              }
              n178 = String To Byte Array(string=w434) -> (unsigned byte array=w413:u8[])
              "mu08ArrayBuf0_3" <- w413
              n179 = case shown="真" w414 {
                tunnel: w413 -> [_ w440]
                frame False {
                }
                frame True {
                  n180 = call "SearchData.vi"("ArrayIn"=w440) -> ("ArrayOut"=w439:u8[])  [unwired: 2 out]
                  "mu08ArrayDatas_3" <- w439
                  n181 = Array Size(array=w439) -> (size(s)=→"mu08ArrayDatasSize_3":i32)
                }
              }
              n182 = Array Size(array=w413) -> (size(s)=→"mu16ArrayBuf0_3":i32)
              n183 = Greater Or Equal?(x=w431, y=u8 4) -> (x >= y?=w429:bool)
              n184 = case shown="假" w429 {
                frame False {
                }
                frame True {
                  n185 = local write "mu08SendCmd_2 2"(u8 0 ("Cmd值")) -> ()
                }
              }
              n186 = local read "写指令_3"() -> (w427:bool)
              n187 = Tick Count (ms)() -> (millisecond timer value=w422:u32)
              n188 = Subtract(x=w422, y=w421) -> (x-y=w420:u32)
            }
          }
          "Time_3" <- w298
          n189 = local read "Start_3"() -> (w295:bool)
          n190 = Not(x=w295) -> (.not. x?=w294:bool)
          n191 = Or(x=w294, y=w292) -> (x .or. y?=w293:bool)
        }
        n192 = VISA Close(VISA resource name=w291, error in (no error)=w290) -> ()  [unwired: 1 out]
      }
    }
  }
  n193 = while {
    stop <- FALSE stop-if-true
    w467 = u16 10 items=["1.0"=10, "1.5"=15, "2.0"=20] ("stop bits (10: 1 bit)")
    n194 = call <vilib>:"Application Directory.vi"() -> ("Application Directory"=w457:path)
    n195 = Path To String(path=w457) -> (string=w456:string)
    n196 = call-poly "VISA Configure Serial Port"("VISA resource name"="1号机端口", "baud rate (9600)"=u32 9600, "data bits (8)"=u16 8, "parity (0:none)"=enum16{"None", "Odd", "Even", "Mark", "Space"}."Even", "stop bits (10: 1 bit)"=w467) -> ("VISA resource name out"=w466:refnum<visa-resource-name>, "error out"=w465:errorcluster)  [unwired: 9 in]
    n197 = Concatenate Strings(w456, "\\TmpDataSave\\ReceiveStrData.xls" ("字符串")) -> (w454:string)
    n198 = String To Path(string=w454) -> (path=w460:path)
    n199 = VISA Flush I/O Buffer(VISA resource name=w466, error in (no error)=w465) -> (VISA resource name out=w464:refnum<visa-resource-name>, error out=w463:errorcluster)  [unwired: 1 in]
    n200 = Open/Create/Replace File(file path (use dialog)=w460, operation (0:open)=T1."open or create" ("操作(0:open)"), access (0:read/write)=enum16{"read/write", "read-only", "write-only"}."read/write" ("权限(0:read/write)")) -> (refnum out=w459:refnum<file>, error out=w458:errorcluster)  [unwired: 3 in, 1 out]
    n201 = flat-sequence {
      tunnel: w458 -> [w498]
      tunnel: w459 -> [w499]
      tunnel: w463 -> [w500]
      tunnel: w464 -> [w501]
      tunnel: [w501] -> w483
      tunnel: [w500] -> w482
      tunnel: [w499] -> w481
      tunnel: [w498] -> w480
      tunnel: [w485] -> w479
      tunnel: [w486] -> w478
      tunnel: [w507] -> w477
      tunnel: [w506] -> w476
      tunnel: [w505] -> w475
      tunnel: [w504] -> w474
      tunnel: [w503] -> w473
      tunnel: [w502] -> w472
      tunnel: w483 -> [w507]
      tunnel: w482 -> [w506]
      tunnel: w481 -> [w505]
      tunnel: w480 -> [w504]
      tunnel: w479 -> [w503]
      tunnel: w478 -> [w502]
      tunnel: w477 -> [w514]
      tunnel: w476 -> [w513]
      tunnel: w475 -> [w512]
      tunnel: w474 -> [w511]
      tunnel: w473 -> [w510]
      tunnel: w472 -> [w509]
      frame #0 {
        n202 = local write "mu08SendCmd"(u8 0 ("Cmd值")) -> ()
        n203 = local write "写指令"(TRUE ("写指令")) -> ()
        n204 = call <vilib>:"Application Directory.vi"() -> ("Application Directory"=w490:path)
        n205 = local write "Start"(FALSE ("Start")) -> ()
        n206 = Path To String(path=w490) -> (string=w491:string)
        n207 = Concatenate Strings(w491, "\\TmpDataSave\\ReceiveNumData.xls" ("字符串")) -> (w493:string)
        n208 = String To Path(string=w493) -> (path=w489:path)
        n209 = Open/Create/Replace File(file path (use dialog)=w489, operation (0:open)=T1."open or create" ("操作(0:open)"), access (0:read/write)=enum16{"read/write", "read-only", "write-only"}."read/write" ("权限(0:read/write)")) -> (refnum out=w486:refnum<file>, error out=w485:errorcluster)  [unwired: 3 in, 1 out]
        "mu08SendCmd" <- u8 0 ("mu08SendCmd")
        "mbfDealData" <- FALSE ("mbfDealData")
      }
      frame #1 {
        n210 = while {
          stop <- "Start" stop-if-true
        }
      }
      frame #2 {
        n211 = while {
          tunnel: w514 -> [w532]
          tunnel: w513 -> [w531]
          tunnel: [w530] -> w517
          tunnel: [w529] -> w516
          shift-right: [w527] -> _
          shift-left: "写指令" -> [w528]
          tunnel: w512 -> [w526]
          tunnel: w511 -> [w525]
          tunnel: w510 -> [w523]
          tunnel: w509 -> [w522]
          stop <- w520 stop-if-true
          n212 = stacked-sequence {
            seq-local: [w546 _ _] -> [_ w586 _]
            seq-local: [w545 _ _] -> [_ w585 _]
            seq-local: [w542 _ _] -> [_ w589 _]
            seq-local: [w533 _ _] -> [_ w573 _]
            seq-local: [w534 _ _] -> [_ w583 _]
            seq-local: [_ w588 _] -> [_ _ w659]
            seq-local: [_ w587 _] -> [_ _ w658]
            seq-local: [_ w584 _] -> [_ _ w649]
            seq-local: [_ w583 _] -> [_ _ w647]
            seq-local: [_ w582 _] -> [_ _ w645]
            seq-local: [_ w577 _] -> [_ _ w638]
            seq-local: [_ w573 _] -> [_ _ w654]
            tunnel: w532 -> [w538 _ _]
            tunnel: w531 -> [w537 _ _]
            tunnel: w528 -> [w544 _ _]
            tunnel: [_ _ w662] -> w530
            tunnel: [_ _ w661] -> w529
            tunnel: [_ _ w653] -> w527
            tunnel: w526 -> [_ _ w651]
            tunnel: w525 -> [_ _ w650]
            tunnel: [_ _ w646] -> w524
            tunnel: w523 -> [_ _ w644]
            tunnel: w522 -> [_ _ w643]
            tunnel: [_ _ w638] -> w521
            frame #0 {
              n213 = VISA Flush I/O Buffer(VISA resource name=w538, error in (no error)=w537) -> (VISA resource name out=w535:refnum<visa-resource-name>, error out=w536:errorcluster)  [unwired: 1 in]
              n214 = case shown="真" w544 {
                tunnel: w538 -> [w560 _]
                tunnel: w537 -> [w559 _]
                tunnel: [w560 w568] -> w546
                tunnel: [w559 w567] -> w545
                tunnel: w536 -> [_ w562]
                tunnel: w535 -> [_ w561]
                frame False {
                }
                frame True {
                  n215 = local read "mu08SendCmd"() -> (w564:u8)
                  n216 = call "SendCmd.vi"("索引 (行)"=w564) -> ("字符串"=w566:string)  [unwired: 1 in]
                  "命令" <- w566
                  n217 = Equal?(x=w564, y=u8 3) -> (x = y?=w563:bool)
                  n218 = case shown="真" w563 {
                    frame False {
                    }
                    frame True {
                      n219 = case shown="真" "mbfUartClearOne" {
                        frame False {
                        }
                        frame True {
                          n220 = local write "mbfUartClearOne"(TRUE ("mbfUartClearOne")) -> ()
                        }
                      }
                    }
                  }
                  n221 = VISA Write(VISA resource name=w561, write buffer=w566, error in (no error)=w562) -> (VISA resource name out=w568:refnum<visa-resource-name>, error out=w567:errorcluster)  [unwired: 1 out]
                }
              }
              n222 = local read "mu08SendCmd"() -> (w541:u8)
              n223 = local read "CmdNumCount"() -> (w543:u8)
              n224 = Equal?(x=w541, y=u8 3) -> (x = y?=w539:bool)
              n225 = case shown="真" w539 {
                frame False {
                  n226 = local write "mbfDealData"(FALSE ("mbfDealData")) -> ()
                }
                frame True {
                  n227 = local write "mbfDealData"(TRUE ("mbfDealData")) -> ()
                }
              }
              n228 = case shown="3" w541 {
                tunnel: [w549 w552 w555 w558] -> w533
                frame 0, Default {
                  n229 = Multiply(x=10, y=2) -> (x*y=w549:i32)
                }
                frame 1 {
                  n230 = Multiply(x=119, y=2) -> (x*y=w552:i32)
                }
                frame 2 {
                  n231 = Multiply(x=30, y=2) -> (x*y=w555:i32)
                }
                frame 3 {
                  n232 = local read "缓冲区数据"() -> (w558:u32)
                }
              }
              n233 = Increment(x=w543) -> (x+1=w542:u8)
              n234 = local write "CmdNumCount"(w542) -> ()
              n235 = Tick Count (ms)() -> (millisecond timer value=w534:u32)
            }
            frame #1 {
              n236 = local read "mu08ArrayDatasSize"() -> (w576:u16)
              n237 = local read "mu16ArrayBuf0"() -> (w581:u16)
              n238 = Greater?(x=w589, y=u8 4) -> (0:w590:bool)
              n239 = Wait (ms)(milliseconds to wait=u32 400 ("等待时间（毫秒）")) -> ()  [unwired: 1 out]
              n240 = Multiply(x=w576, y=u8 2) -> (x*y=w574:u16)
              n241 = local read "mbfDealData"() -> (w580:bool)
              n242 = call "WWorWD.vi"("strModelChoice"="strModelChoice") -> ("WWorWD"=w571:bool)  [unwired: 9 in, 1 out]
              n243 = Equal?(x=w574, y=w581) -> (x = y?=w579:bool)
              n244 = And(x=w579, y=w580) -> (x .and. y?=w578:bool)
              n245 = case shown="真" w578 {
                selector: w578 -> [_ w597]
                tunnel: [w594 w615] -> w584
                tunnel: [w594 w610] -> w582
                tunnel: [FALSE w602] -> w577
                tunnel: w571 -> [_ w598]
                frame False {
                  w594 = string[] []
                }
                frame True {
                  w606 = u32 0 ("y")
                  # "TotalRemainTime = 0\n&& StepRemainTime = 0"
                  n246 = local read "mu08ArrayDatas"() -> (w601:u8[])
                  n247 = case shown="真" w598 {
                    tunnel: [w623 w629] -> w595
                    tunnel: [w622 w628] -> w596
                    tunnel: w601 -> [w621 w627]
                    tunnel: [18 ("索引") 20 ("索引")] -> w600
                    tunnel: [19 ("索引") 21 ("索引")] -> w599
                    tunnel: w597 -> [w618 w624]
                    frame False {
                      # "WW"
                      n248 = call "DealData.vi"("mbfDealData"=w618, "ArrayIn"=w621) -> ("mu08BufSize"=w622:u8, "Result"=w623:string[])
                    }
                    frame True {
                      # "WD"
                      n249 = call "WD_DealData.vi"("mbfDealData"=w624, "ArrayIn"=w627) -> ("ResultArrayOut"=w629:string[], "mu08BufSize"=w628:u8)
                    }
                  }
                  "mu08BufSize" <- w596
                  n250 = property on="strResultArrayOut" class="Arr (严格)"("Value"=w595) -> ()  [unwired: 2 in, 2 out]
                  n251 = call "GetDataFromString.vi"("strArrayIn"=w595) -> ("strArrayBuf"=w609:string[], "mu32ArrayOut"=w608:u32[])
                  n252 = Index Array(array=w608, index #1=w600, index #2=w599) -> (element #1=w607:u32, element #2=w605:u32)
                  n253 = Equal?(x=w607, y=w606) -> (x = y?=w604:bool)
                  n254 = Equal?(x=w606, y=w605) -> (x = y?=w603:bool)
                  n255 = Get Date/Time String(want seconds? (F)=TRUE ("需要秒？(F)")) -> (time string=w616:string)  [unwired: 2 in, 1 out]
                  n256 = Get Date/Time String(want seconds? (F)=TRUE ("需要秒？(F)")) -> (time string=w612:string)  [unwired: 2 in, 1 out]
                  n257 = And(x=w604, y=w603) -> (x .and. y?=w602:bool)
                  n258 = Insert Into Array(array=w595, index=0 ("索引"), new element=w616) -> (w615:string[])
                  n259 = Insert Into Array(array=w609, index=0 ("索引"), new element=w612) -> (w610:string[])
                }
              }
              n260 = case shown="真" w590 {
                tunnel: [w631 w635] -> w588
                tunnel: [w630 w634] -> w587
                tunnel: w586 -> [w631 w635]
                tunnel: w585 -> [w630 w634]
                frame False {
                  n261 = local write "写指令"(FALSE ("写指令")) -> ()
                }
                frame True {
                  n262 = local write "mu08SendCmd"(u8 3 ("mu08SendCmd")) -> ()
                  n263 = local write "CmdNumCount"(u8 0 ("CmdNumCount")) -> ()
                  n264 = local write "写指令"(TRUE ("写指令")) -> ()
                }
              }
            }
            frame #2 {
              n265 = property class="Instr"(reference=w659, error in=w658) -> (reference out=w664:refnum<visa-resource-name>, error out=w663:errorcluster, "Bytes at Port"=w641:u32)
              "缓冲区数据" <- w641
              n266 = VISA Read(VISA resource name=w664, byte count=w654, error in (no error)=w663) -> (VISA resource name out=w662:refnum<visa-resource-name>, read buffer=w660:string, error out=w661:errorcluster)  [unwired: 1 out]
              n267 = Greater?(x=w641, y=250) -> (0:w640:bool)
              n268 = local read "mu08SendCmd"() -> (w657:u8)
              n269 = case shown="真" w640 {
                tunnel: w651 -> [_ w675]
                tunnel: w650 -> [_ w674]
                tunnel: w649 -> [_ w673]
                tunnel: w645 -> [_ w672]
                tunnel: w644 -> [_ w669]
                tunnel: w643 -> [_ w668]
                frame False {
                }
                frame True {
                  n270 = Array To Spreadsheet String(array=w673, 3:"%s" ("格式字符串")) -> (spreadsheet string=w677:string)  [unwired: 1 in]
                  n271 = Array To Spreadsheet String(array=w672, 3:"%s" ("格式字符串")) -> (spreadsheet string=w670:string)  [unwired: 1 in]
                  n272 = Write to Text File(file (use dialog)=w675, text=w677, error in=w674) -> ()  [unwired: 1 in, 3 out]
                  n273 = Write to Text File(file (use dialog)=w668, text=w670, error in=w669) -> ()  [unwired: 1 in, 3 out]
                }
              }
              n274 = String To Byte Array(string=w660) -> (unsigned byte array=w639:u8[])
              "mu08ArrayBuf0" <- w639
              n275 = case shown="真" w640 {
                tunnel: w639 -> [_ w666]
                frame False {
                }
                frame True {
                  n276 = call "SearchData.vi"("ArrayIn"=w666) -> ("ArrayOut"=w665:u8[])  [unwired: 2 out]
                  "mu08ArrayDatas" <- w665
                  n277 = Array Size(array=w665) -> (size(s)=→"mu08ArrayDatasSize":i32)
                }
              }
              n278 = Array Size(array=w639) -> (size(s)=→"mu16ArrayBuf0":i32)
              n279 = Greater Or Equal?(x=w657, y=u8 4) -> (x >= y?=w655:bool)
              n280 = case shown="假" w655 {
                frame False {
                }
                frame True {
                  n281 = local write "mu08SendCmd"(u8 0 ("Cmd值")) -> ()
                }
              }
              n282 = Tick Count (ms)() -> (millisecond timer value=w648:u32)
              n283 = local read "写指令"() -> (w653:bool)
              n284 = Subtract(x=w648, y=w647) -> (x-y=w646:u32)
            }
          }
          "Time" <- w524
          n285 = local read "Start"() -> (w519:bool)
          n286 = Not(x=w519) -> (.not. x?=w518:bool)
          n287 = Or(x=w518, y=w521) -> (x .or. y?=w520:bool)
        }
        n288 = VISA Close(VISA resource name=w517, error in (no error)=w516) -> ()  [unwired: 1 out]
      }
    }
  }
  n289 = while {
    stop <- FALSE stop-if-true
    w693 = u16 10 items=["1.0"=10, "1.5"=15, "2.0"=20] ("stop bits (10: 1 bit)")
    n290 = call <vilib>:"Application Directory.vi"() -> ("Application Directory"=w683:path)
    n291 = Path To String(path=w683) -> (string=w682:string)
    n292 = Concatenate Strings(w682, "\\TmpDataSave\\ReceiveStrData4.xls" ("字符串")) -> (w680:string)
    n293 = call-poly "VISA Configure Serial Port"("VISA resource name"="4号机端口", "baud rate (9600)"=u32 9600, "data bits (8)"=u16 8, "parity (0:none)"=enum16{"None", "Odd", "Even", "Mark", "Space"}."Even", "stop bits (10: 1 bit)"=w693) -> ("VISA resource name out"=w692:refnum<visa-resource-name>, "error out"=w691:errorcluster)  [unwired: 9 in]
    n294 = String To Path(string=w680) -> (path=w686:path)
    n295 = VISA Flush I/O Buffer(VISA resource name=w692, error in (no error)=w691) -> (VISA resource name out=w690:refnum<visa-resource-name>, error out=w689:errorcluster)  [unwired: 1 in]
    n296 = Open/Create/Replace File(file path (use dialog)=w686, operation (0:open)=T1."open or create" ("操作(0:open)"), access (0:read/write)=enum16{"read/write", "read-only", "write-only"}."read/write" ("权限(0:read/write)")) -> (refnum out=w685:refnum<file>, error out=w684:errorcluster)  [unwired: 3 in, 1 out]
    n297 = flat-sequence {
      tunnel: w684 -> [w724]
      tunnel: w685 -> [w725]
      tunnel: w689 -> [w726]
      tunnel: w690 -> [w727]
      tunnel: [w727] -> w709
      tunnel: [w726] -> w708
      tunnel: [w725] -> w707
      tunnel: [w724] -> w706
      tunnel: [w710] -> w705
      tunnel: [w711] -> w704
      tunnel: [w733] -> w703
      tunnel: [w732] -> w702
      tunnel: [w731] -> w701
      tunnel: [w730] -> w700
      tunnel: [w729] -> w699
      tunnel: [w728] -> w698
      tunnel: w709 -> [w733]
      tunnel: w708 -> [w732]
      tunnel: w707 -> [w731]
      tunnel: w706 -> [w730]
      tunnel: w705 -> [w729]
      tunnel: w704 -> [w728]
      tunnel: w703 -> [w740]
      tunnel: w702 -> [w739]
      tunnel: w701 -> [w738]
      tunnel: w700 -> [w737]
      tunnel: w699 -> [w736]
      tunnel: w698 -> [w735]
      frame #0 {
        n298 = call <vilib>:"Application Directory.vi"() -> ("Application Directory"=w715:path)
        n299 = Path To String(path=w715) -> (string=w716:string)
        n300 = local write "mu08SendCmd_4"(u8 0 ("Cmd值")) -> ()
        n301 = local write "写指令_4"(TRUE ("写指令")) -> ()
        n302 = local write "Start_4"(FALSE ("Start_4")) -> ()
        n303 = Concatenate Strings(w716, "\\TmpDataSave\\ReceiveNumData4.xls" ("字符串")) -> (w718:string)
        n304 = String To Path(string=w718) -> (path=w714:path)
        n305 = Open/Create/Replace File(file path (use dialog)=w714, operation (0:open)=T1."open or create" ("操作(0:open)"), access (0:read/write)=enum16{"read/write", "read-only", "write-only"}."read/write" ("权限(0:read/write)")) -> (refnum out=w711:refnum<file>, error out=w710:errorcluster)  [unwired: 3 in, 1 out]
        "mu08SendCmd_4" <- u8 0 ("mu08SendCmd")
        "mbfDealData_4" <- FALSE ("mbfDealData")
      }
      frame #1 {
        n306 = while {
          stop <- "Start_4" stop-if-true
        }
      }
      frame #2 {
        n307 = while {
          tunnel: w740 -> [w758]
          tunnel: w739 -> [w757]
          tunnel: [w756] -> w743
          tunnel: [w755] -> w742
          shift-right: [w753] -> _
          shift-left: "写指令_4" -> [w754]
          tunnel: w738 -> [w752]
          tunnel: w737 -> [w751]
          tunnel: w736 -> [w749]
          tunnel: w735 -> [w748]
          stop <- w745 stop-if-true
          n308 = stacked-sequence {
            seq-local: [w772 _ _] -> [_ w812 _]
            seq-local: [w771 _ _] -> [_ w811 _]
            seq-local: [w768 _ _] -> [_ w815 _]
            seq-local: [w759 _ _] -> [_ w799 _]
            seq-local: [w760 _ _] -> [_ w809 _]
            seq-local: [_ w814 _] -> [_ _ w885]
            seq-local: [_ w813 _] -> [_ _ w884]
            seq-local: [_ w810 _] -> [_ _ w875]
            seq-local: [_ w809 _] -> [_ _ w873]
            seq-local: [_ w808 _] -> [_ _ w871]
            seq-local: [_ w803 _] -> [_ _ w864]
            seq-local: [_ w799 _] -> [_ _ w880]
            tunnel: w758 -> [w764 _ _]
            tunnel: w757 -> [w763 _ _]
            tunnel: w754 -> [w770 _ _]
            tunnel: [_ _ w888] -> w756
            tunnel: [_ _ w887] -> w755
            tunnel: [_ _ w879] -> w753
            tunnel: w752 -> [_ _ w877]
            tunnel: w751 -> [_ _ w876]
            tunnel: [_ _ w872] -> w750
            tunnel: w749 -> [_ _ w870]
            tunnel: w748 -> [_ _ w869]
            tunnel: [_ _ w864] -> w744
            frame #0 {
              n309 = VISA Flush I/O Buffer(VISA resource name=w764, error in (no error)=w763) -> (VISA resource name out=w761:refnum<visa-resource-name>, error out=w762:errorcluster)  [unwired: 1 in]
              n310 = case shown="真" w770 {
                tunnel: w764 -> [w786 _]
                tunnel: w763 -> [w785 _]
                tunnel: [w786 w794] -> w772
                tunnel: [w785 w793] -> w771
                tunnel: w762 -> [_ w788]
                tunnel: w761 -> [_ w787]
                frame False {
                }
                frame True {
                  n311 = local read "mu08SendCmd_4"() -> (w790:u8)
                  n312 = call "SendCmd.vi"("索引 (行)"=w790) -> ("字符串"=w792:string)  [unwired: 1 in]
                  "命令_4" <- w792
                  n313 = Equal?(x=w790, y=u8 3) -> (x = y?=w789:bool)
                  n314 = case shown="真" w789 {
                    frame False {
                    }
                    frame True {
                      n315 = case shown="真" "mbfUartClearOne_4" {
                        frame False {
                        }
                        frame True {
                          n316 = local write "mbfUartClearOne_4"(TRUE ("mbfUartClearOne")) -> ()
                        }
                      }
                    }
                  }
                  n317 = VISA Write(VISA resource name=w787, write buffer=w792, error in (no error)=w788) -> (VISA resource name out=w794:refnum<visa-resource-name>, error out=w793:errorcluster)  [unwired: 1 out]
                }
              }
              n318 = local read "mu08SendCmd_4"() -> (w767:u8)
              n319 = local read "CmdNumCount_4"() -> (w769:u8)
              n320 = Equal?(x=w767, y=u8 3) -> (x = y?=w765:bool)
              n321 = case shown="真" w765 {
                frame False {
                  n322 = local write "mbfDealData_4"(FALSE ("mbfDealData")) -> ()
                }
                frame True {
                  n323 = local write "mbfDealData_4"(TRUE ("mbfDealData")) -> ()
                }
              }
              n324 = case shown="3" w767 {
                tunnel: [w775 w778 w781 w784] -> w759
                frame 0, Default {
                  n325 = Multiply(x=10, y=2) -> (x*y=w775:i32)
                }
                frame 1 {
                  n326 = Multiply(x=119, y=2) -> (x*y=w778:i32)
                }
                frame 2 {
                  n327 = Multiply(x=30, y=2) -> (x*y=w781:i32)
                }
                frame 3 {
                  n328 = local read "缓冲区数据_4"() -> (w784:u32)
                }
              }
              n329 = Increment(x=w769) -> (x+1=w768:u8)
              n330 = local write "CmdNumCount_4"(w768) -> ()
              n331 = Tick Count (ms)() -> (millisecond timer value=w760:u32)
            }
            frame #1 {
              n332 = local read "mu08ArrayDatasSize_4"() -> (w802:u16)
              n333 = local read "mu16ArrayBuf0_4"() -> (w807:u16)
              n334 = Greater?(x=w815, y=u8 4) -> (0:w816:bool)
              n335 = Wait (ms)(milliseconds to wait=u32 400 ("等待时间（毫秒）")) -> ()  [unwired: 1 out]
              n336 = Multiply(x=w802, y=u8 2) -> (x*y=w800:u16)
              n337 = local read "mbfDealData_4"() -> (w806:bool)
              n338 = call "WWorWD.vi"("strModelChoice"="strModelChoice_4") -> ("WWorWD"=w797:bool)  [unwired: 9 in, 1 out]
              n339 = Equal?(x=w800, y=w807) -> (x = y?=w805:bool)
              n340 = And(x=w805, y=w806) -> (x .and. y?=w804:bool)
              n341 = case shown="真" w804 {
                selector: w804 -> [_ w823]
                tunnel: [w820 w841] -> w810
                tunnel: [w820 w836] -> w808
                tunnel: [FALSE w828] -> w803
                tunnel: w797 -> [_ w824]
                frame False {
                  w820 = string[] []
                }
                frame True {
                  w832 = u32 0 ("y")
                  # "TotalRemainTime = 0\n&& StepRemainTime = 0"
                  n342 = local read "mu08ArrayDatas_4"() -> (w827:u8[])
                  n343 = case shown="真" w824 {
                    tunnel: [w849 w855] -> w821
                    tunnel: [w848 w854] -> w822
                    tunnel: w827 -> [w847 w853]
                    tunnel: [18 ("索引") 20 ("索引")] -> w826
                    tunnel: [19 ("索引") 21 ("索引")] -> w825
                    tunnel: w823 -> [w844 w850]
                    frame False {
                      # "WW"
                      n344 = call "DealData.vi"("mbfDealData"=w844, "ArrayIn"=w847) -> ("mu08BufSize"=w848:u8, "Result"=w849:string[])
                    }
                    frame True {
                      # "WD"
                      n345 = call "WD_DealData.vi"("mbfDealData"=w850, "ArrayIn"=w853) -> ("ResultArrayOut"=w855:string[], "mu08BufSize"=w854:u8)
                    }
                  }
                  "mu08BufSize_4" <- w822
                  n346 = property on="strResultArrayOut_4" class="Arr (严格)"("Value"=w821) -> ()  [unwired: 2 in, 2 out]
                  n347 = call "GetDataFromString.vi"("strArrayIn"=w821) -> ("strArrayBuf"=w835:string[], "mu32ArrayOut"=w834:u32[])
                  n348 = Index Array(array=w834, index #1=w826, index #2=w825) -> (element #1=w833:u32, element #2=w831:u32)
                  n349 = Equal?(x=w833, y=w832) -> (x = y?=w830:bool)
                  n350 = Equal?(x=w832, y=w831) -> (x = y?=w829:bool)
                  n351 = Get Date/Time String(want seconds? (F)=TRUE ("需要秒？(F)")) -> (time string=w842:string)  [unwired: 2 in, 1 out]
                  n352 = Get Date/Time String(want seconds? (F)=TRUE ("需要秒？(F)")) -> (time string=w838:string)  [unwired: 2 in, 1 out]
                  n353 = And(x=w830, y=w829) -> (x .and. y?=w828:bool)
                  n354 = Insert Into Array(array=w821, index=0 ("索引"), new element=w842) -> (w841:string[])
                  n355 = Insert Into Array(array=w835, index=0 ("索引"), new element=w838) -> (w836:string[])
                }
              }
              n356 = case shown="真" w816 {
                tunnel: [w857 w861] -> w814
                tunnel: [w856 w860] -> w813
                tunnel: w812 -> [w857 w861]
                tunnel: w811 -> [w856 w860]
                frame False {
                  n357 = local write "写指令_4"(FALSE ("写指令")) -> ()
                }
                frame True {
                  n358 = local write "mu08SendCmd_4"(u8 3 ("mu08SendCmd")) -> ()
                  n359 = local write "CmdNumCount_4"(u8 0 ("CmdNumCount")) -> ()
                  n360 = local write "写指令_4"(TRUE ("写指令")) -> ()
                }
              }
            }
            frame #2 {
              n361 = property class="Instr"(reference=w885, error in=w884) -> (reference out=w890:refnum<visa-resource-name>, error out=w889:errorcluster, "Bytes at Port"=w867:u32)
              "缓冲区数据_4" <- w867
              n362 = VISA Read(VISA resource name=w890, byte count=w880, error in (no error)=w889) -> (VISA resource name out=w888:refnum<visa-resource-name>, read buffer=w886:string, error out=w887:errorcluster)  [unwired: 1 out]
              n363 = Greater?(x=w867, y=250) -> (0:w866:bool)
              n364 = local read "mu08SendCmd_4"() -> (w883:u8)
              n365 = case shown="真" w866 {
                tunnel: w877 -> [_ w901]
                tunnel: w876 -> [_ w900]
                tunnel: w875 -> [_ w899]
                tunnel: w871 -> [_ w898]
                tunnel: w870 -> [_ w895]
                tunnel: w869 -> [_ w894]
                frame False {
                }
                frame True {
                  n366 = Array To Spreadsheet String(array=w899, 3:"%s" ("格式字符串")) -> (spreadsheet string=w903:string)  [unwired: 1 in]
                  n367 = Array To Spreadsheet String(array=w898, 3:"%s" ("格式字符串")) -> (spreadsheet string=w896:string)  [unwired: 1 in]
                  n368 = Write to Text File(file (use dialog)=w901, text=w903, error in=w900) -> ()  [unwired: 1 in, 3 out]
                  n369 = Write to Text File(file (use dialog)=w894, text=w896, error in=w895) -> ()  [unwired: 1 in, 3 out]
                }
              }
              n370 = String To Byte Array(string=w886) -> (unsigned byte array=w865:u8[])
              "mu08ArrayBuf0_4" <- w865
              n371 = case shown="真" w866 {
                tunnel: w865 -> [_ w892]
                frame False {
                }
                frame True {
                  n372 = call "SearchData.vi"("ArrayIn"=w892) -> ("ArrayOut"=w891:u8[])  [unwired: 2 out]
                  "mu08ArrayDatas_4" <- w891
                  n373 = Array Size(array=w891) -> (size(s)=→"mu08ArrayDatasSize_4":i32)
                }
              }
              n374 = Array Size(array=w865) -> (size(s)=→"mu16ArrayBuf0_4":i32)
              n375 = Greater Or Equal?(x=w883, y=u8 4) -> (x >= y?=w881:bool)
              n376 = case shown="假" w881 {
                frame False {
                }
                frame True {
                  n377 = local write "mu08SendCmd_4"(u8 0 ("Cmd值")) -> ()
                }
              }
              n378 = local read "写指令_4"() -> (w879:bool)
              n379 = Tick Count (ms)() -> (millisecond timer value=w874:u32)
              n380 = Subtract(x=w874, y=w873) -> (x-y=w872:u32)
            }
          }
          "Time_4" <- w750
          n381 = local read "Start_4"() -> (w747:bool)
          n382 = Not(x=w747) -> (.not. x?=w746:bool)
          n383 = Or(x=w746, y=w744) -> (x .or. y?=w745:bool)
        }
        n384 = VISA Close(VISA resource name=w743, error in (no error)=w742) -> ()  [unwired: 1 out]
      }
    }
  }
